vi "read data.vi"(11 "Analyze Msg in":refnum<class "Analyze Msg.lvclass">) -> (2 "Image Nr.":i32, 3 "Image":T1)   [LabVIEW 2014, in "Analyze Actor.lvlib" / "Analyze Msg.lvclass"]
uses:
  Analyze Msg.lvclass
  <vilib>/vision/Image Controls.llb/IMAQ Image.ctl
  Analyze Msg.lvclass/Analyze Msg.ctl
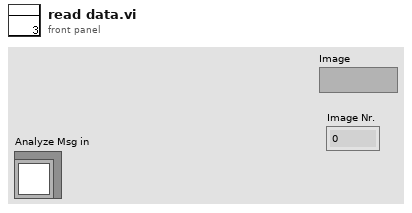
[diagram p1: front panel]
types:
  T1 = typedef "IMAQ Image.ctl" = refnum<image>
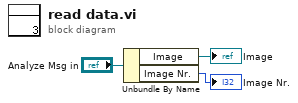
[diagram p0: block diagram]
diagram:
  n1 = Unbundle By Name("Analyze Msg in") -> ("Image"=→"Image":T1, "Image Nr."=→"Image Nr.":i32)
